vi "modbus2.vi"(8 "error out":errorcluster, 9 "TCP Connection Refnum in":refnum<k5>, 10 "Quantity":u16, 11 "Starting Address":u16) -> (0 "error out 2":errorcluster, 2 "TCP Connection Refnum (dup)":refnum<k5>, 3 "Slave Input Registers":u16[](array[numeric]) caption="Slave Input Registers (Read Only)")   [LabVIEW 2017]
uses:
  monitor/Source Code/VIs/Modbus/Modbus VIs.llb/MB Modbus Command.ctl
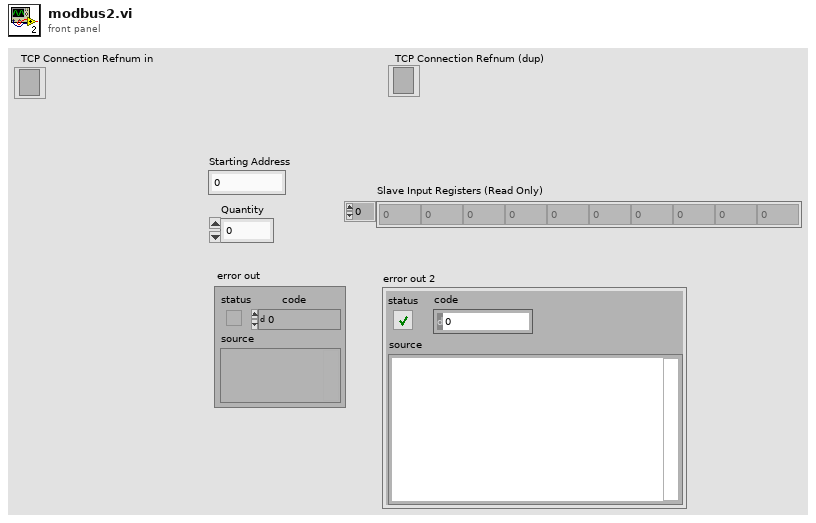
[diagram p1: front panel]
types:
  T1 = typedef "MB Modbus Command.ctl" = cluster{"Function Code":u8, "Starting Address":u16, "Quantity":u16, "Data":u16[], "Discrete":bool[]}
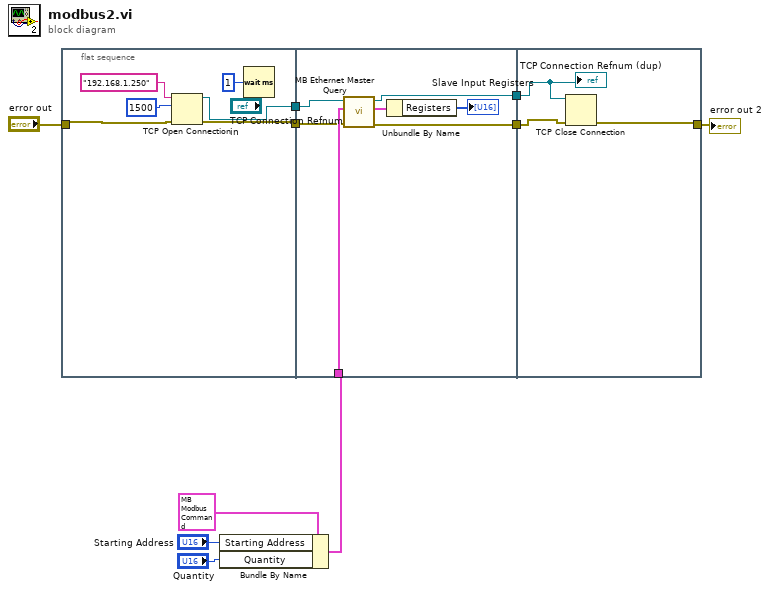
[diagram p0: block diagram]
diagram:
  n1 = flat-sequence {
    tunnel: "error out" -> [w13]
    tunnel: [w11] -> w2
    tunnel: [w12] -> w1
    tunnel: [w21] -> w10
    tunnel: [w20] -> w9
    tunnel: w6 -> [w19]
    tunnel: w2 -> [w18]
    tunnel: w1 -> [w17]
    tunnel: w10 -> [w26]
    tunnel: w9 -> [w25]
    tunnel: [w24] -> w3
    frame #0 {
      n2 = TCP Open Connection(address="192.168.1.250" ("Remote IP Address"), remote port or service name=u16 1500 ("Remote Port"), error in (no error)=w13) -> (connection ID=w11:refnum<k5>, error out=w12:errorcluster)  [unwired: 2 in]
      n3 = Wait (ms)(milliseconds to wait=u32 1) -> ()  [unwired: 1 out]
    }
    frame #1 {
      n4 = call "MB Ethernet Master Query.vi"("error in (no error)"=w17, "Modbus Command"=w19, "TCP Connection Refnum in"=w18) -> ("error out"=w20:errorcluster, "Registers"=w22:cluster{"Registers":u16[], "Discrete":bool[]}, "TCP Connection Refnum (dup)"=w21:refnum<k5>)  [unwired: 4 in, 2 out]
      n5 = Unbundle By Name(w22) -> ("Registers"=→"Slave Input Registers":u16[])
    }
    frame #2 {
      n6 = TCP Close Connection(connection ID=w26, error in (no error)=w25) -> (error out=w24:errorcluster)  [unwired: 1 in, 1 out]
      "TCP Connection Refnum (dup)" <- w26
    }
  }
  n7 = Bundle By Name(cluster=T1 {"Function Code"=3, "Starting Address"=1000, "Quantity"=20, "Data"=[], "Discrete"=[FALSE, TRUE, TRUE, TRUE, FALSE, FALSE, FALSE, FALSE, FALSE, TRUE]} ("MODBUS Command 2"), "Starting Address"="Starting Address", "Quantity"="Quantity") -> (w6:T1)
  "error out 2" <- w3
